vi "Extract Measurement Parameters.vi"(8 "error in (no error)":errorcluster, 11 "Measurement Parameters":refnum<class "String Database.lvclass">[](array[class])) -> (0 "error out":errorcluster, 2 "RF Calibration Parameters":T1[](array[typedef]))   [LabVIEW 2018, in "niRFSTS Sequence Flow.lvclass"]
uses:
  niRFSTS Sequence Flow.lvclass
  Plugins/String Database.lvlibp/String Database.lvclass
  Typedefs/RF Calibration Parameters.ctl
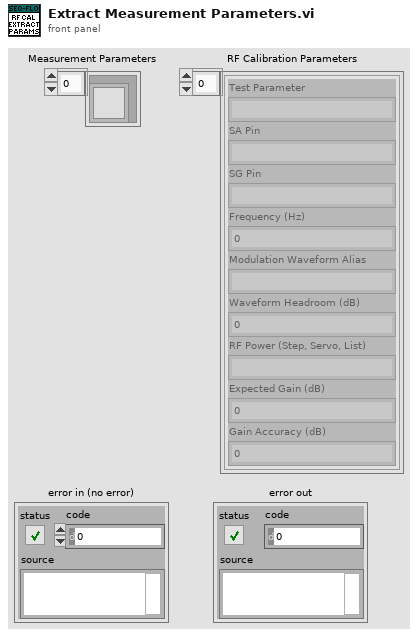
[diagram p1: front panel]
types:
  T1 = typedef "niRFSTS Sequence Flow.lvclass/RF Calibration Parameters.ctl" = cluster{"Test Parameter":string, "SA Pin":string, "SG Pin":string, "Frequency (Hz)":dbl, "Modulation Waveform Alias":string, "Waveform Headroom (dB)":dbl, "RF Power (Step, Servo, List)":string, "Expected Gain (dB)":dbl, "Gain Accuracy (dB)":dbl}
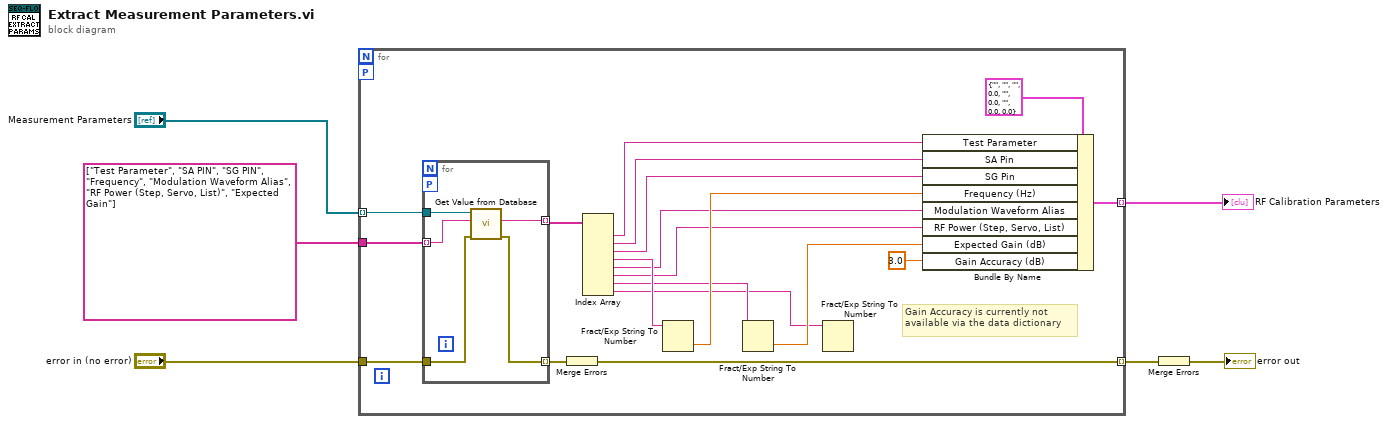
[diagram p0: block diagram]
diagram:
  n1 = for {
    tunnel: "Measurement Parameters" -> [w10] mode=indexing
    tunnel: string[] ["Test Parameter", "SA PIN", "SG PIN", "Frequency", "Modulation Waveform Alias", "RF Power (Step, Servo, List)", "Expected Gain"] -> [w25]
    tunnel: "error in (no error)" -> [w24]
    tunnel: [w22] -> w5 mode=indexing
    workers-P: _ -> [_]
    tunnel: [w12] -> w1 mode=indexing
    # "Gain Accuracy is currently not available via the data dictionary"
    n2 = for {
      tunnel: w10 -> [w30]
      tunnel: w25 -> [w29] mode=indexing
      tunnel: [w26] -> w20 mode=indexing
      tunnel: w24 -> [w28]
      tunnel: [w27] -> w23 mode=indexing
      workers-P: _ -> [_]
      n3 = call "Get Value from Database.vi"("error in (no error)"=w28, "Entry Name"=w29, "Message in"=w30) -> ("error out"=w27:errorcluster, "Entry Value"=w26:string)  [unwired: 5 in, 2 out]
    }
    n4 = Merge Errors(w23) -> (w22:errorcluster)
    n5 = Index Array(array=w20) -> (element #1=w19:string, element #2=w18:string, element #3=w17:string, element #4=w16:string, element #5=w14:string, element #6=w9:string, element #7=w8:string, element #8=w7:string)  [unwired: 8 in]
    n6 = Fract/Exp String To Number(string=w16) -> (number=w15:dbl)  [unwired: 3 in, 1 out]
    n7 = Fract/Exp String To Number(string=w8) -> (number=w13:dbl)  [unwired: 3 in, 1 out]
    n8 = Fract/Exp String To Number(string=w7) -> ()  [unwired: 3 in, 2 out]
    n9 = Bundle By Name(cluster=T1 {"Test Parameter"="", "SA Pin"="", "SG Pin"="", "Frequency (Hz)"=0.0, "Modulation Waveform Alias"="", "Waveform Headroom (dB)"=0.0, "RF Power (Step, Servo, List)"="", "Expected Gain (dB)"=0.0, "Gain Accuracy (dB)"=0.0} ("RF Calibration Parameters"), "Test Parameter"=w19, "SA Pin"=w18, "SG Pin"=w17, "Frequency (Hz)"=w15, "Modulation Waveform Alias"=w14, "RF Power (Step, Servo, List)"=w9, "Expected Gain (dB)"=w13, "Gain Accuracy (dB)"=3.0) -> (w12:T1)
  }
  "RF Calibration Parameters" <- w1
  n10 = Merge Errors(w5) -> (→"error out":errorcluster)
